vi "Open.vi"(8 "error in (no error)":errorcluster, 10 "Path":path, 11 "Controller in":refnum<class "Controller.lvclass">) -> (0 "error out":errorcluster, 3 "Controller out":refnum<class "Controller.lvclass">)   [LabVIEW 2013, in "SET Project Editor.lvlib" / "Controller.lvclass"]
uses:
  Controller.lvclass
  Controller.lvclass/Controller.ctl
  SET Project Data/Project Data Class/Project Data.lvclass
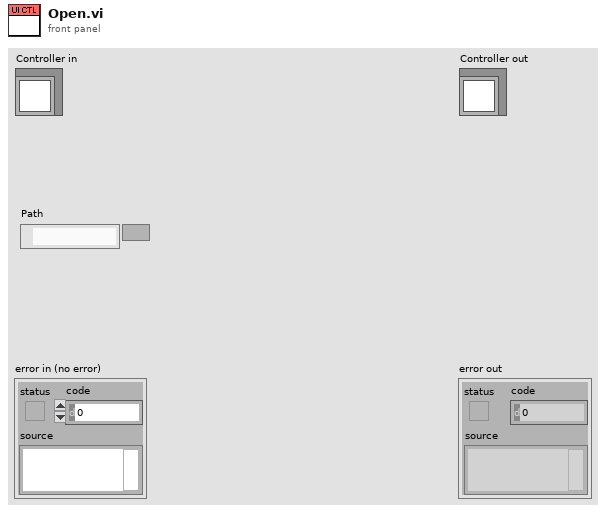
[diagram p1: front panel]
types:
  T1 = enum16{"Left Button", "Center Button", "Right Button", "Window Close"}
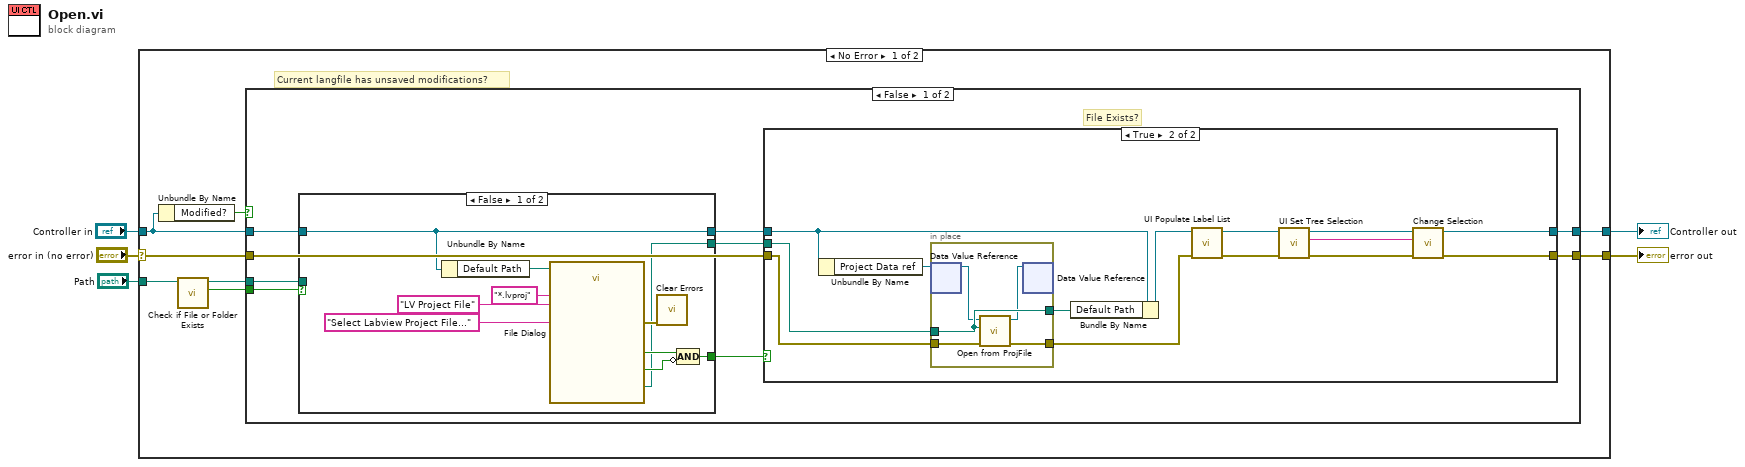
[diagram p0: block diagram]
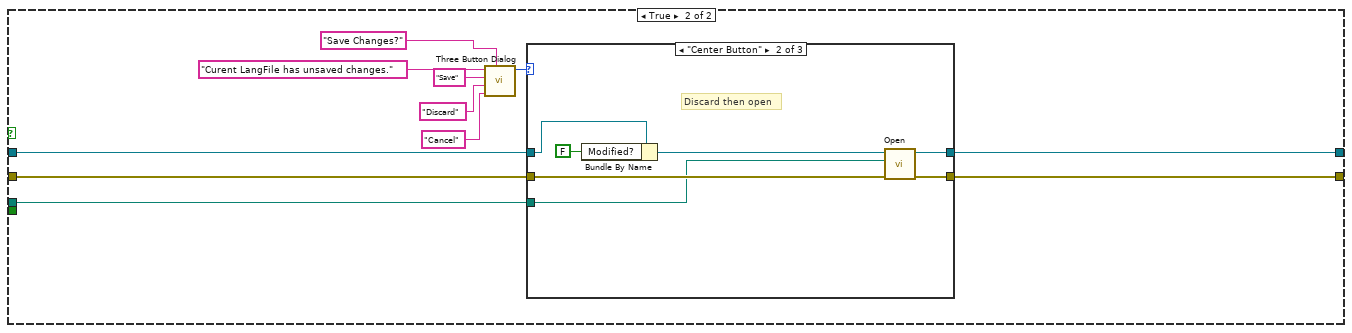
[diagram p4: hidden frame]
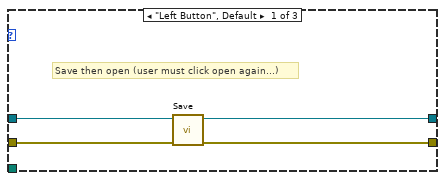
[diagram p5: hidden frame]
diagram:
  n1 = case shown="No Error" "error in (no error)" {
    selector: "error in (no error)" -> [w10 w82]
    tunnel: [w9 w82] -> w4
    tunnel: [w11 w81] -> w2
    tunnel: "Controller in" -> [w12 w81]
    tunnel: "Path" -> [w8 _]
    frame No Error {
      # "Current langfile has unsaved modifications?"
      n2 = Unbundle By Name(w12) -> ("Modified?"=w13:bool)
      n3 = call <vilib>:"Check if File or Folder Exists.vi"("path"=w8) -> ("file or folder exists?"=w7:bool, "dup path"=w6:path)  [unwired: 8 in, 1 out]
      n4 = case shown="False" w13 {
        tunnel: w10 -> [w22 w59]
        tunnel: [w21 w60] -> w11
        tunnel: [w20 w58] -> w9
        tunnel: w12 -> [w17 w67]
        tunnel: w7 -> [w16 _]
        tunnel: w6 -> [w15 w57]
        frame False {
          # "File Exists?"
          n5 = case shown="False" w16 {
            selector: w16 -> [_ w33]
            tunnel: [w27 w34] -> w19
            tunnel: [w26 w33] -> w18
            tunnel: w17 -> [w23 w35]
            tunnel: w15 -> [_ w34]
            tunnel: [w23 w35] -> w14
            frame False {
              n6 = Unbundle By Name(w23) -> ("Default Path"=w25:path)
              n7 = call "File Dialog"("start path"=w25, "prompt"="Select Labview Project File...", "pattern (all files)"="*.lvproj", "pattern label"="LV Project File") -> ("selected path"=w27:path, "exists"=w30:bool, "cancelled"=w29:bool, "error out"=w28:errorcluster)  [unwired: 8 in]
              n8 = call <vilib>:"Clear Errors.vi"("error in (no error)"=w28) -> ()  [unwired: 6 in, 1 out]
              n9 = Compound Arithmetic op=AND(w30, invert w29) -> (w26:bool)
            }
            frame True {
            }
          }
          n10 = case shown="True" w18 {
            tunnel: w14 -> [w37 w48]
            tunnel: w22 -> [w36 w51]
            tunnel: [w37 w39] -> w21
            tunnel: [w36 w38] -> w20
            tunnel: w19 -> [_ w50]
            frame False {
            }
            frame True {
              n11 = Unbundle By Name(w48) -> ("Project Data ref"=w47:refnum<data-value>)
              n12 = in-place {
                in-place-border: w51 -> [w56]
                in-place-border: [w55] -> w45
                in-place-border: w50 -> [w54]
                in-place-border: [w54] -> w49
                n13 = in-place-dvr #1(w47) -> (w53:refnum<class "Project Data.lvclass">)  [unwired: 1 out]
                n14 = call "Open from ProjFile.vi"("error in (no error)"=w56, "LV Project file path"=w54, "LanguageData in"=w53) -> ("error out"=w55:errorcluster, "LanguageData out"=w52:refnum<class "Project Data.lvclass">)  [unwired: 7 in]
                n15 = in-place-dvr #1(w52) -> ()  [unwired: 2 out]
              }
              n16 = Bundle By Name(cluster=w48, "Default Path"=w49) -> (w46:refnum<class "Controller.lvclass">)
              n17 = call-dynamic "UI Populate Label List.vi"("error in (no error)"=w45, "Controller in"=w46) -> ("error out"=w43:errorcluster, "Controller out"=w44:refnum<class "Controller.lvclass">)  [unwired: 8 in]
              n18 = call-dynamic "UI Set Tree Selection.vi"("error in (no error)"=w43, "Controller in"=w44) -> ("error out"=w40:errorcluster, "Tag out"=w41:string, "Controller out"=w42:refnum<class "Controller.lvclass">)  [unwired: 7 in]
              n19 = call-dynamic "Change Selection.vi"("error in (no error)"=w40, "UID"=w41, "Controller in"=w42) -> ("error out"=w38:errorcluster, "Controller out"=w39:refnum<class "Controller.lvclass">)  [unwired: 7 in]
            }
          }
        }
        frame True {
          n20 = call <vilib>:"Three Button Dialog.vi"("Window Title (\"\")"="Save Changes?" ("Window Title (\"\")"), "Right Button Text (\"Cancel\")"="Cancel" ("Right Button Text (\"Cancel\")"), "Center Button Text (\"No\")"="Discard" ("Center Button Text (\"No\")"), "Left Button Text (\"Yes\")"="Save" ("Left Button Text (\"Yes\")"), "message"="Curent LangFile has unsaved changes.") -> ("Which Button?"=w61:T1)  [unwired: 6 in]
          n21 = case shown="\"Center Button\"" w61 {
            tunnel: w67 -> [w71 w78 w80]
            tunnel: [w70 w75 w80] -> w60
            tunnel: w59 -> [w69 w74 w79]
            tunnel: [w68 w73 w79] -> w58
            tunnel: w57 -> [_ w72 _]
            frame "Left Button", Default {
              # "Save then open (user must click open again...)"
              n22 = call-dynamic "Save.vi"("error in (no error)"=w69, "Controller in"=w71) -> ("error out"=w68:errorcluster, "Controller out"=w70:refnum<class "Controller.lvclass">)  [unwired: 8 in]
            }
            frame "Center Button" {
              # "Discard then open"
              n23 = Bundle By Name(cluster=w78, "Modified?"=FALSE) -> (w76:refnum<class "Controller.lvclass">)
              n24 = call-dynamic "Open.vi"("error in (no error)"=w74, "Path"=w72, "Controller in"=w76) -> ("error out"=w73:errorcluster, "Controller out"=w75:refnum<class "Controller.lvclass">)  [unwired: 7 in]
            }
            frame "Right Button" {
              # "Cancel"
            }
          }
        }
      }
    }
    frame Error {
    }
  }
  "error out" <- w4
  "Controller out" <- w2
